vi "Create_Default_Dest.vi"(8 "error in (no error)":errorcluster, 10 "project name":string, 11 "Class in":refnum<class "Installer.lvclass">) -> (0 "error out":errorcluster, 3 "Class out":refnum<class "Installer.lvclass">)   [LabVIEW 2020, in "Installer.lvclass"]
uses:
  <vilib>/AppBuilder/IB_Classes/Installer/Installer.lvclass
  <vilib>/AppBuilder/IB_Classes/Installer/Installer.lvclass/Installer.ctl
  <vilib>/AppBuilder/IB_Classes/Destination/userFolder/userFolder.lvclass
  <vilib>/AppBuilder/IB_Classes/Destination/IB_Destination.lvclass
  <resource>/Framework/Providers/Builds/Installer/CDK_GLOBAL_LABELS.vi
  e:/builds/penguin/labview/branches/2020/dev/dist/vi.lib/AppBuilder/IB_Classes/Destination/IB_Destination.lvclass
  e:/builds/penguin/labview/branches/2020/dev/dist/vi.lib/AppBuilder/IB_Classes/Destination/userFolder/userFolder.lvclass
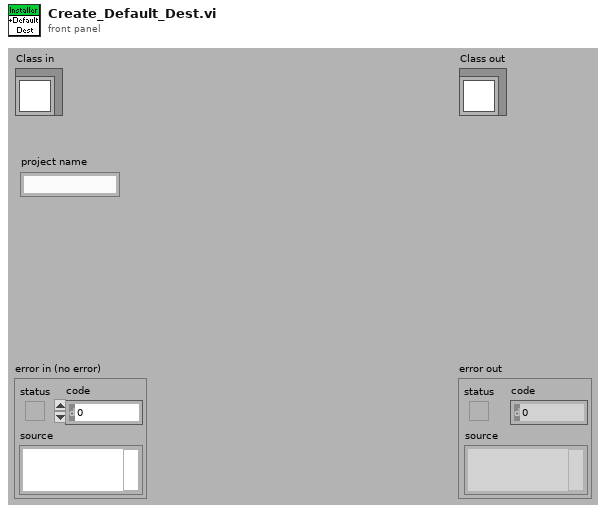
[diagram p1: front panel]
types:
  T1 = typedef "CDK_sTypeDef_AppBitness.ctl" = enum16{"invalid", "32-bit", "64-bit"}
  T2 = typedef "IB_Destination.ctl" = cluster{"name":string, "unlock":bool, "parentTag":string, "destTag":string, "eng_installPath":string}
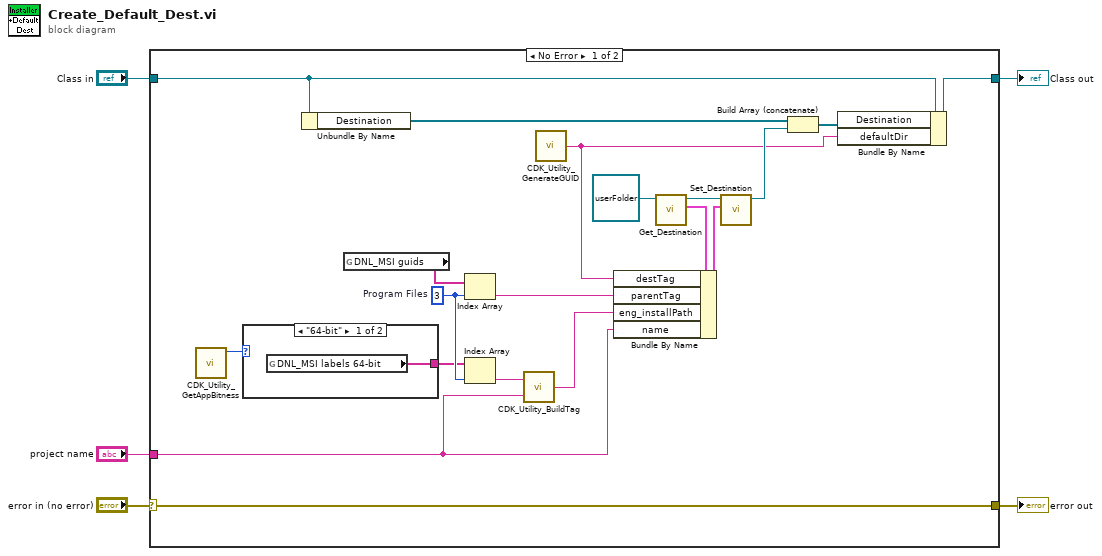
[diagram p0: block diagram]
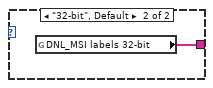
[diagram p2: hidden frame]
diagram:
  n1 = case shown="No Error" "error in (no error)" {
    selector: "error in (no error)" -> [w6 w28]
    tunnel: [w6 w28] -> w4
    tunnel: [w22 w27] -> w2
    tunnel: "Class in" -> [w23 w27]
    tunnel: "project name" -> [w7 _]
    frame No Error {
      w12 = 3  # Program Files
      n2 = call <resource>:"CDK_Utility_GetAppBitness.vi"() -> ("app bitness"=w8:T1)  [unwired: 11 out]
      n3 = case shown="\"64-bit\"" w8 {
        tunnel: [w25 w26] -> w9
        frame "64-bit" {
          n4 = global read "CDK_GLOBAL_LABELS.vi" "DNL_MSI labels 64-bit"() -> (w25:string[])
        }
        frame "32-bit", Default {
          n5 = global read "CDK_GLOBAL_LABELS.vi" "DNL_MSI labels 32-bit"() -> (w26:string[])
        }
      }
      n6 = Unbundle By Name(w23) -> ("Destination"=w19:refnum<class "IB_Destination.lvclass">[])
      n7 = global read "CDK_GLOBAL_LABELS.vi" "DNL_MSI guids"() -> (w15:string[])
      n8 = Index Array(array=w15, index=w12) -> (element=w14:string)
      n9 = Index Array(array=w9, index=w12) -> (element=w11:string)
      n10 = call <resource>:"CDK_Utility_BuildTag.vi"("name or relative path"=w7, "BasePath"=w11) -> ("appended path"=w10:string)
      n11 = call <resource>:"CDK_Utility_GenerateGUID.vi"() -> ("GUID"=w13:string)  [unwired: 9 out]
      n12 = call <vilib>:"Get_Destination.vi"("IB_Destination in"=refnum<class "userFolder.lvclass"> refnum ("IB_Dest_Stnd.lvclass")) -> ("data"=w16:T2, "IB_Destination out"=w17:refnum<class "userFolder.lvclass">)  [unwired: 1 in, 8 out]
      n13 = Bundle By Name(cluster=w16, "destTag"=w13, "parentTag"=w14, "eng_installPath"=w10, "name"=w7) -> (w24:T2)
      n14 = call <vilib>:"Set_Destination.vi"("data"=w24, "IB_Destination in"=w17) -> ("IB_Destination out"=w21:refnum<class "userFolder.lvclass">)  [unwired: 1 in, 8 out]
      n15 = Build Array (concatenate)(w19, w21) -> (w20:refnum<class "IB_Destination.lvclass">[])
      n16 = Bundle By Name(cluster=w23, "Destination"=w20, "defaultDir"=w13) -> (w22:refnum<class "Installer.lvclass">)
    }
    frame Error {
    }
  }
  "error out" <- w4
  "Class out" <- w2
